vi "EminemNetworking.vi"(8 "error in (no error)":errorcluster) -> (0 "error out":errorcluster)   [LabVIEW 2023]
uses:
  <vilib>/Rock Robotics/Network Tables/NT Write Boolean.vi
  EminemGlobals.vi
  <vilib>/Rock Robotics/Network Tables/NT Write Number.vi
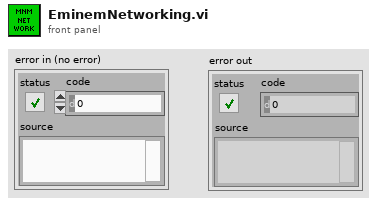
[diagram p1: front panel]
types:
  T1 = typedef "EminemStatesEnum.ctl" = enum16{"0-Init", "1-WaitForCmd", "2-Cancel", "3-ShootStart", "4-ShootRev", "5-ShootUpToSpd?", "6-ShootStartFeed&Timer", "7-ShootTimerOrSensorDone", "8-ShootDone", "9-AmpStart", "10-AmpUpToSpd?", "11-AmpStartFeed&Timer", "12-AmpTimerOrSensorDone", "13-AmpDone"}
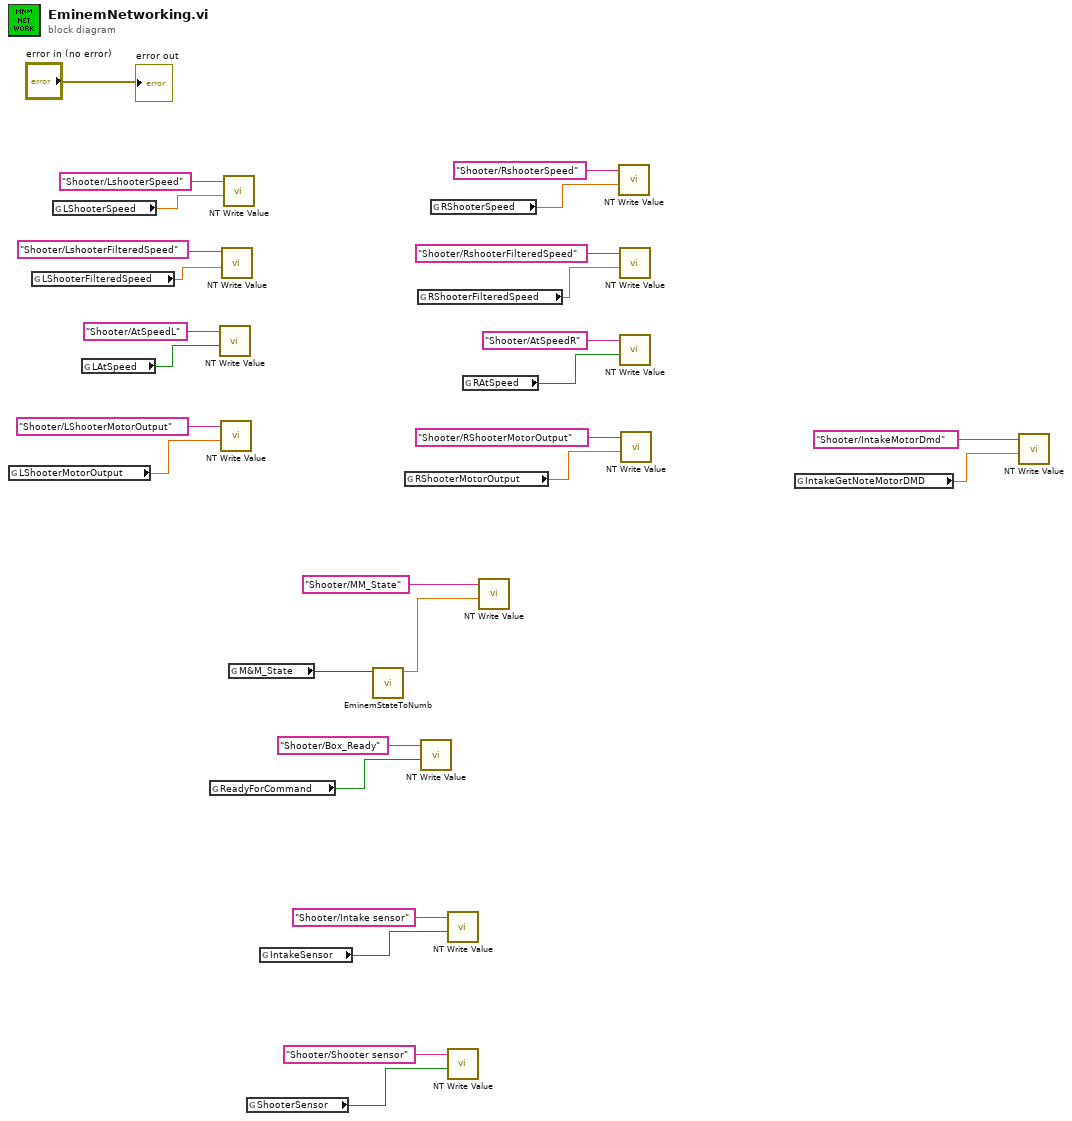
[diagram p0: block diagram]
diagram:
  n1 = global read "EminemGlobals.vi" "LShooterMotorOutput"() -> (w10:dbl)
  n2 = global read "EminemGlobals.vi" "LShooterFilteredSpeed"() -> (w16:dbl)
  n3 = global read "EminemGlobals.vi" "LShooterSpeed"() -> (w15:dbl)
  n4 = global read "EminemGlobals.vi" "LAtSpeed"() -> (w14:bool)
  n5 = global read "EminemGlobals.vi" "ReadyForCommand"() -> (w8:bool)
  n6 = call-poly <vilib>:"NT Write Value.vi"("value"=w14, "name"="Shooter/AtSpeedL") -> ()  [unwired: 9 in, 1 out]
  n7 = call-poly <vilib>:"NT Write Value.vi"("value"=w10, "name"="Shooter/LShooterMotorOutput") -> ()  [unwired: 9 in, 1 out]
  n8 = call-poly <vilib>:"NT Write Value.vi"("value"=w16, "name"="Shooter/LshooterFilteredSpeed") -> ()  [unwired: 9 in, 1 out]
  n9 = call-poly <vilib>:"NT Write Value.vi"("value"=w15, "name"="Shooter/LshooterSpeed") -> ()  [unwired: 9 in, 1 out]
  n10 = global read "EminemGlobals.vi" "M&M_State"() -> (w3:T1)
  n11 = global read "EminemGlobals.vi" "ShooterSensor"() -> (w7:bool)
  n12 = global read "EminemGlobals.vi" "IntakeSensor"() -> (w6:bool)
  n13 = call "EminemStateToNumb.vi"("Eminim_state"=w3) -> ("StateNumber"=w1:dbl)  [unwired: 10 in]
  n14 = global read "EminemGlobals.vi" "RShooterMotorOutput"() -> (w9:dbl)
  n15 = global read "EminemGlobals.vi" "RShooterFilteredSpeed"() -> (w12:dbl)
  n16 = call-poly <vilib>:"NT Write Value.vi"("value"=w8, "name"="Shooter/Box_Ready") -> ()  [unwired: 9 in, 1 out]
  n17 = global read "EminemGlobals.vi" "RShooterSpeed"() -> (w13:dbl)
  n18 = call-poly <vilib>:"NT Write Value.vi"("value"=w6, "name"="Shooter/Intake sensor") -> ()  [unwired: 9 in, 1 out]
  n19 = call-poly <vilib>:"NT Write Value.vi"("value"=w7, "name"="Shooter/Shooter sensor") -> ()  [unwired: 9 in, 1 out]
  n20 = global read "EminemGlobals.vi" "RAtSpeed"() -> (w11:bool)
  n21 = call-poly <vilib>:"NT Write Value.vi"("value"=w1, "name"="Shooter/MM_State") -> ()  [unwired: 9 in, 1 out]
  n22 = call-poly <vilib>:"NT Write Value.vi"("value"=w13, "name"="Shooter/RshooterSpeed") -> ()  [unwired: 9 in, 1 out]
  n23 = call-poly <vilib>:"NT Write Value.vi"("value"=w12, "name"="Shooter/RshooterFilteredSpeed") -> ()  [unwired: 9 in, 1 out]
  n24 = call-poly <vilib>:"NT Write Value.vi"("value"=w11, "name"="Shooter/AtSpeedR") -> ()  [unwired: 9 in, 1 out]
  n25 = call-poly <vilib>:"NT Write Value.vi"("value"=w9, "name"="Shooter/RShooterMotorOutput") -> ()  [unwired: 9 in, 1 out]
  n26 = global read "EminemGlobals.vi" "IntakeGetNoteMotorDMD"() -> (w4:dbl)
  n27 = call-poly <vilib>:"NT Write Value.vi"("value"=w4, "name"="Shooter/IntakeMotorDmd") -> ()  [unwired: 9 in, 1 out]
  "error out" <- "error in (no error)"
